vi "Read trigger level  (0.0 V).vi"(8 "error in (no error)":errorcluster, 11 "Configure Edge Trigger Source Msg in":refnum<class "Configure Edge Trigger Source Msg.lvclass">) -> (0 "error out":errorcluster, 2 "trigger level  (0.0 V)":dbl[unit] format="%.3f", 3 "Configure Edge Trigger Source Msg out":refnum<class "Configure Edge Trigger Source Msg.lvclass">)   [LabVIEW 2016, in "CS++Scope.lvlib" / "Configure Edge Trigger Source Msg.lvclass"]
uses:
  Configure Edge Trigger Source Msg.lvclass
  Configure Edge Trigger Source Msg.lvclass/Configure Edge Trigger Source Msg.ctl
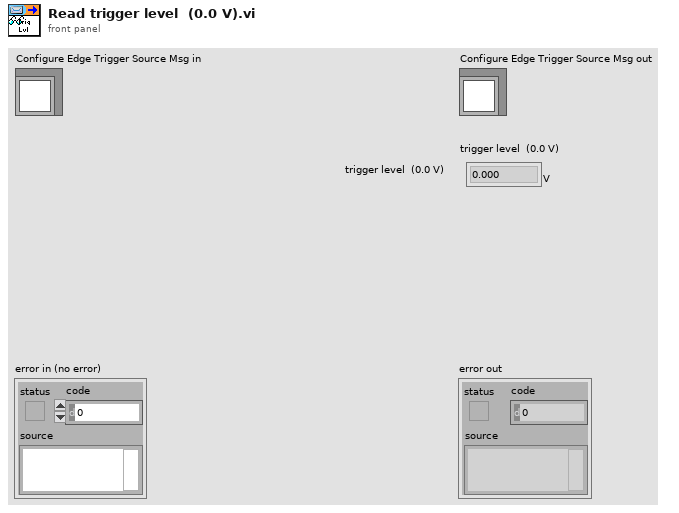
[diagram p1: front panel]
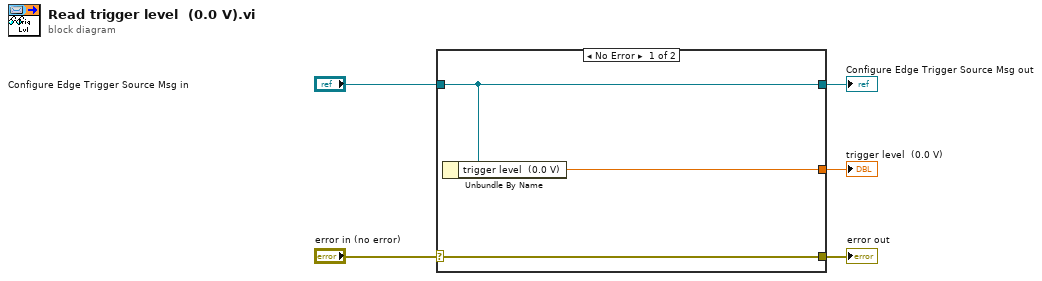
[diagram p0: block diagram]
diagram:
  n1 = case shown="No Error" "error in (no error)" {
    selector: "error in (no error)" -> [w8 w9]
    tunnel: [w8 w9] -> w4
    tunnel: [w7 w10] -> w2
    tunnel: "Configure Edge Trigger Source Msg in" -> [w7 w10]
    tunnel: [w6 _] -> w1
    frame No Error {
      n2 = Unbundle By Name(w7) -> ("trigger level  (0.0 V)"=w6:dbl[unit])
    }
    frame Error {
    }
  }
  "error out" <- w4
  "Configure Edge Trigger Source Msg out" <- w2
  "trigger level  (0.0 V)" <- w1
